vi "Read and Write Controls to Config File.vi"(7 "Action":T1, 8 "error in":errorcluster, 10 "Control References":refnum<vi>[](array[refnum]), 11 "Configuration File Reference In":T2) -> (0 "error out":errorcluster, 3 "Configuration File Reference Out":T2)   [LabVIEW 2018]
doc: "Writes the values of an array of controls to a configuration file or reads them back.\n<b>Control References</b> is an array of the references of the controls to be saved.\n\nThe section name is the name of the VI that holds the control.\nThe key name is the label of the control."
uses:
  <vilib>/Utility/config.llb/Config Data RefNum.ctl
  Load and Save Controls_LV2009.llb/RWC_Actions.ctl
  <vilib>/Utility/config.llb/Read Key (String).vi
  <vilib>/Utility/config.llb/Write Key (String).vi
  <vilib>/Utility/config.llb/NI_LVConfig.lvlib
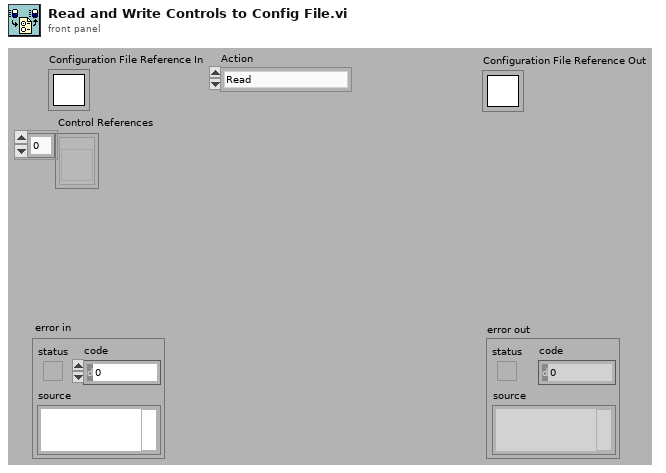
[diagram p1: front panel]
types:
  T1 = typedef "RWC_Actions.ctl" = enum16{"Read", "Write", "Read and Create"}
  T2 = typedef "NI_LVConfig.lvlib/Config Data RefNum.ctl" = refnum<k1>
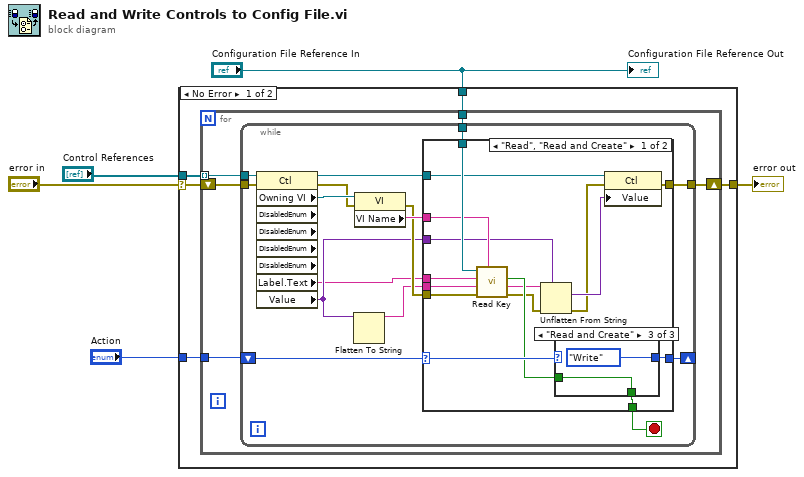
[diagram p0: block diagram]
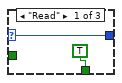
[diagram p2: hidden frame]
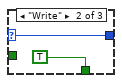
[diagram p3: hidden frame]
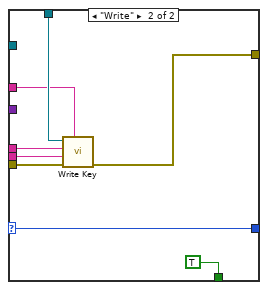
[diagram p4: hidden frame]
diagram:
  n1 = case shown="No Error" "error in" {
    selector: "error in" -> [w7 w61]
    tunnel: "Control References" -> [w10 _]
    tunnel: [w9 w61] -> w4
    tunnel: "Configuration File Reference In" -> [w8 _]
    tunnel: "Action" -> [w6 _]
    frame No Error {
      n2 = for {
        tunnel: w10 -> [w15] mode=indexing
        shift-right: [w13] -> w9
        shift-left: w7 -> [w14]
        tunnel: w8 -> [w12]
        tunnel: w6 -> [w11]
        n3 = while {
          tunnel: w15 -> [w30]
          tunnel: w14 -> [w29]
          tunnel: [w28] -> w13
          tunnel: w12 -> [w27]
          shift-right: [w19] -> _
          shift-left: w11 -> [w20]
          stop <- w21 stop-if-true
          n4 = property class="Ctl" props=["Owning VI", "DisabledEnum", "DisabledEnum", "DisabledEnum", "DisabledEnum", "Label", "Text", "Value"](reference=w30, error in=w29) -> (reference out=w22:refnum<vi>, error out=w24:errorcluster, "Owning VI"=w26:refnum<vi>, "Label.Text"=w16:string, "Value"=w17:variant)  [unwired: 4 out]
          n5 = Flatten To String(anything=w17) -> (data string=w18:string)  [unwired: 3 in, 2 out]
          n6 = property class="VI"(reference=w26, error in=w24) -> (error out=w23:errorcluster, "VI Name"=w25:string)  [unwired: 1 out]
          n7 = case shown="\"Read\", \"Read and Create\"" w20 {
            selector: w20 -> [w41 w54]
            tunnel: [w42 w60] -> w28
            tunnel: w27 -> [w44 w59]
            tunnel: w25 -> [w37 w58]
            tunnel: w16 -> [w45 w57]
            tunnel: w23 -> [w46 w56]
            tunnel: w22 -> [w43 _]
            tunnel: [w40 TRUE] -> w21
            tunnel: [w39 w54] -> w19
            tunnel: w18 -> [w36 w53]
            tunnel: w17 -> [w34 _]
            frame "Read", "Read and Create" {
              n8 = call-poly <vilib>:"Read Key.vi"("section"=w37, "error in (no error)"=w46, "default value"=w36, "key"=w45, "refnum"=w44) -> ("error out"=w32:errorcluster, "value"=w35:string, "found?"=w38:bool)  [unwired: 3 in, 1 out]
              n9 = Unflatten From String(type=w34, binary string=w35, error in (no error)=w32) -> (value=w33:variant, error out=w31:errorcluster)  [unwired: 2 in, 1 out]
              n10 = case shown="\"Read and Create\"" w41 {
                selector: w41 -> [w48 w49 _]
                tunnel: [TRUE ("found?") TRUE w52] -> w40
                tunnel: [w48 w49 RWC_Actions."Write"] -> w39
                tunnel: w38 -> [_ _ w52]
                frame "Read" {
                }
                frame "Write" {
                }
                frame "Read and Create" {
                }
              }
              n11 = property class="Ctl"(reference=w43, error in=w31, "Value"=w33) -> (error out=w42:errorcluster)  [unwired: 1 out]
            }
            frame "Write" {
              n12 = call-poly <vilib>:"Write Key.vi"("section"=w58, "error in (no error)"=w56, "value"=w53, "key"=w57, "refnum"=w59) -> ("error out"=w60:errorcluster)  [unwired: 4 in, 2 out]
            }
          }
        }
      }
    }
    frame Error {
    }
  }
  "error out" <- w4
  "Configuration File Reference Out" <- "Configuration File Reference In"
